vi "wait on reply.vi"(8 "error in":errorcluster {"code" format="Error %.0f"}, 10 "timeout in ms (-1)":i32=-1, 11 "NATS Subscriber in":refnum<class "NATS Subscription.lvclass">) -> (0 "error out":errorcluster {"code" format="Error %.0f"}, 2 "time out":bool, 3 "nats message":T1)   [LabVIEW 2024, in "NAT Subscription.lvlib" / "NATS Subscription.lvclass"]
uses:
  NATS Subscription.lvclass
  Controls/nats message.ctl
  Controls/msg type.ctl
  NATS Subscription.lvclass/NATS Subscription.ctl
  get reply queue.vi
  NATS Core.lvlib
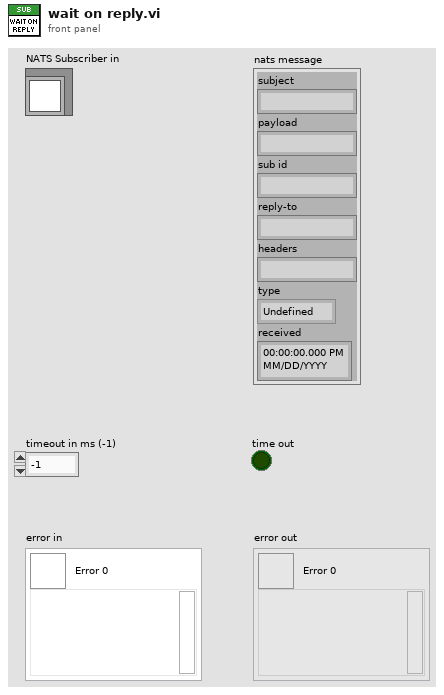
[diagram p1: front panel]
types:
  T1 = typedef "NATS Core.lvlib/nats message.ctl" = cluster{"subject":string, "payload":string, "sub id":string, "reply-to":string, "headers":string, "type":T2, "received":timestamp}
  T2 = typedef "NATS Core.lvlib/msg type.ctl" = enum16{"Undefined", "MSG", "HMSG", "+OK", "PING", "PONG", "-ERR", "INFO"}
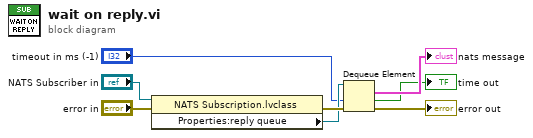
[diagram p0: block diagram]
diagram:
  n1 = property class="NATS Subscription.lvclass"(reference="NATS Subscriber in", error in="error in") -> (error out=w8:errorcluster, "Properties:reply queue"=w5:refnum<queue>)  [unwired: 1 out]
  n2 = Dequeue Element(queue=w5, timeout in ms (-1)="timeout in ms (-1)", error in (no error)=w8) -> (element=→"nats message":T1, timed out?=→"time out":bool, error out=→"error out":errorcluster)  [unwired: 1 out]
